vi "Z_ROI_compiler.vi"(7 "dISABLE":bool=TRUE, 8 "error in (no error)":errorcluster, 10 "Acquired z-plane index / volume index":i32, 11 "AOL_Globals":T2={"Imaging Protocol"=enum."AOL Z-Stack", "Number of POI"=0, "Number of Miniscans"=0, "Number of Trials"=0, "Number of Cycles "=0, "# Averaged Frames"=0, "Laser power (%)"=0, "Pockels"=0.0, "Acquisition Length (sec)"=0.0, "Fill time (us)"=0.0, "POI Dwell time (us)"=0.0, "Miniscan Dwell time per pixel (us)"=0.0, "PMT 1"=0.0, "PMT 2"=0.0, "Back Apperture"=200.0, "Frame Size"=0, "Center Frequency"=0.0, "Field of View"=0.0, "DwellTime (us)"=0.0, "Wavelength (nm)"=0.0, "Zoom"=0.0, "AOL Z"=0.0, "AOL Mode"=enum."Raster", "GridXY"=0.0, "GridZ"=0.0, "TriggerPeriod (sec)"=0.0, "Number of Pixels in Miniscan"=0, "Experiment folder path"=path "", "X centre"=0.0, "Y centre"=0.0, "Angle (degrees)"=0.0, "Plane Mode"=0, "Threshold"=[], "Regenerate Chirps"=FALSE, "Rectangle ROI length (pixels)"=0, "Rectangle ROI height (pixels)"=0, "AOD fill"=0, "Samples Wait after Trigger"=0, "StartUp Delay"=0, "Slip Cycle"=163840, "Add Cycle"=FALSE} {"Plane Mode" items=["XY Plane"]; "Frame Size" items=["100X100"=100, "128X128"=128, "200X200"=200, "256X256"=256, "512X512"=512, "1024x1024"=1024, "2048x2048"=2048]; "Back Apperture" format="%#.6g"; "Pockels" format="%#.6g"; "PMT 2" format="%#.6g"; "PMT 1" format="%#.6g"; "Angle (degrees)" format="%#.6g"; "POI Dwell time (us)" format="%#.6g"}) -> (0 "error out":errorcluster, 1 "AOL_Globals":T2={"Imaging Protocol"=enum."AOL Z-Stack", "Number of POI"=0, "Number of Miniscans"=0, "Number of Trials"=0, "Number of Cycles "=0, "# Averaged Frames"=0, "Laser power (%)"=0, "Pockels"=0.0, "Acquisition Length (sec)"=0.0, "Fill time (us)"=0.0, "POI Dwell time (us)"=0.0, "Miniscan Dwell time per pixel (us)"=0.0, "PMT 1"=0.0, "PMT 2"=0.0, "Back Apperture"=200.0, "Frame Size"=0, "Center Frequency"=0.0, "Field of View"=0.0, "DwellTime (us)"=0.0, "Wavelength (nm)"=0.0, "Zoom"=0.0, "AOL Z"=0.0, "AOL Mode"=enum."Raster", "GridXY"=0.0, "GridZ"=0.0, "TriggerPeriod (sec)"=0.0, "Number of Pixels in Miniscan"=0, "Experiment folder path"=path "", "X centre"=0.0, "Y centre"=0.0, "Angle (degrees)"=0.0, "Plane Mode"=0, "Threshold"=[], "Regenerate Chirps"=FALSE, "Rectangle ROI length (pixels)"=0, "Rectangle ROI height (pixels)"=0, "AOD fill"=0, "Samples Wait after Trigger"=0, "StartUp Delay"=0, "Slip Cycle"=163840, "Add Cycle"=FALSE} {"Plane Mode" items=["XY Plane"]; "Frame Size" items=["100X100"=100, "128X128"=128, "200X200"=200, "256X256"=256, "512X512"=512, "1024x1024"=1024, "2048x2048"=2048]; "Back Apperture" format="%#.6g"; "Pockels" format="%#.6g"; "PMT 2" format="%#.6g"; "PMT 1" format="%#.6g"; "Angle (degrees)" format="%#.6g"; "POI Dwell time (us)" format="%#.6g"}, 2 "ROI Coordinates (broken down to miniscans)":T7, 3 "Cycle time (us)":dbl, 4 "ROI Attributes (broken down to miniscans)":T1[](array[typedef]) {"ROI group ID" format="%#_6f"; "Laser Power (%)" format="%#_6f"; "Zoom" format="%#_6f"; "Frame Size" format="%#_6f"; "Number of lines" format="%#_6f"; "Composite ID" format="%#_6f"; "Angle (deg)" format="%#_6f"; "ROI Time (ns)" format="%#_6f"; "ROI ID" format="%#_6f"; "Pixels in ROI" format="%#_6f"; "ROI index" format="%#_6f"; "Z stop" format="%#_6f"; "Y stop" format="%#_6f"; "X stop" format="%#_6f"; "Z start" format="%#_6f"; "X start" format="%#_6f"; "Y start" format="%#_6f"}, 5 "Zoom":dbl[](array[numeric]), 6 "NO ROI AVAILABLE!!!":bool)   [LabVIEW 2013]
uses:
  Typedefs/ROI XY coordinates cluster.ctl
  Typedefs/Controls/AOL_Globals.ctl
  Typedefs/Imaging Protocols enum.ctl
  Typedefs/Frame Size.ctl
  Typedefs/AOL modes.ctl
  Typedefs/Plane Mode.ctl
  User Interface/Visualisation/Functional Imaging Viewer/Typedefs/ROI parameters data type.ctl
  User Interface/Visualisation/Functional Imaging Viewer/SubVIs/Experiment header interface/Typedefs/Save-Load-Save as-Load last enum.ctl
  User Interface/Visualisation/Functional Imaging Viewer/SubVIs/Experiment header interface/Typedefs/Header file type enum.ctl
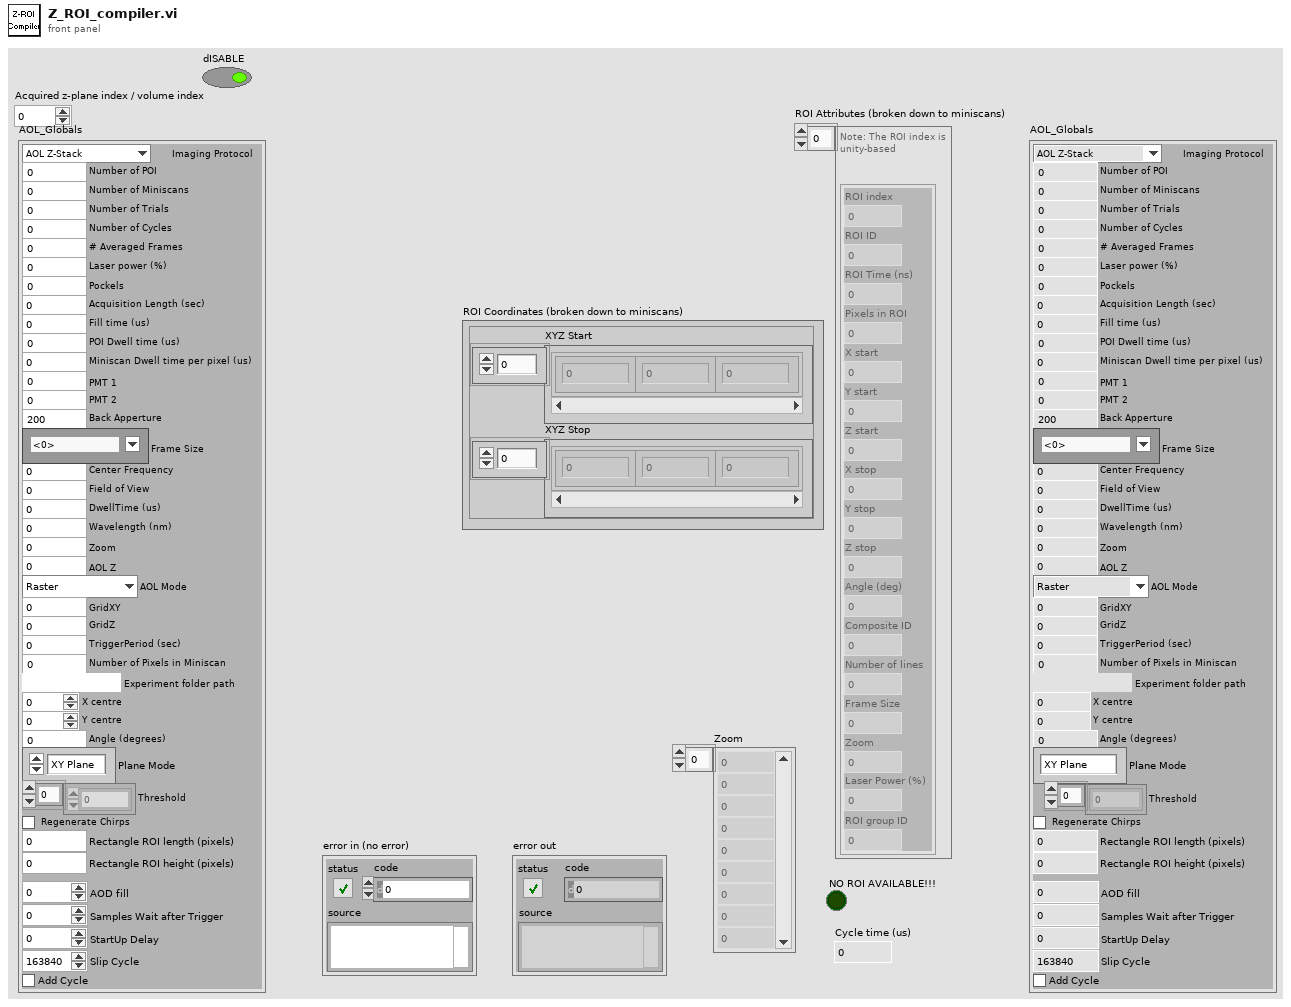
[diagram p1: front panel]
types:
  T1 = typedef "ROI parameters data type.ctl" = cluster{"ROI index":dbl, "ROI ID":dbl, "ROI Time (ns)":dbl, "Pixels in ROI":dbl, "X start":dbl, "Y start":dbl, "Z start":dbl, "X stop":dbl, "Y stop":dbl, "Z stop":dbl, "Angle (deg)":dbl, "Composite ID":dbl, "Number of lines":dbl, "Frame Size":dbl, "Zoom":dbl, "Laser Power (%)":dbl, "ROI group ID":dbl}
  T2 = typedef "AOL_Globals.ctl" = cluster{"Imaging Protocol":T3, "Number of POI":u16, "Number of Miniscans":u16, "Number of Trials":u16, "Number of Cycles ":u64, "# Averaged Frames":u16, "Laser power (%)":u8, "Pockels":dbl, "Acquisition Length (sec)":dbl, "Fill time (us)":dbl, "POI Dwell time (us)":dbl, "Miniscan Dwell time per pixel (us)":dbl, "PMT 1":dbl, "PMT 2":dbl, "Back Apperture":dbl, "Frame Size":T4, "Center Frequency":dbl, "Field of View":dbl, "DwellTime (us)":dbl, "Wavelength (nm)":dbl, "Zoom":dbl, "AOL Z":dbl, "AOL Mode":T5, "GridXY":dbl, "GridZ":dbl, "TriggerPeriod (sec)":dbl, "Number of Pixels in Miniscan":u16, "Experiment folder path":path, "X centre":dbl, "Y centre":dbl, "Angle (degrees)":dbl, "Plane Mode":T6, "Threshold":u16[], "Regenerate Chirps":bool, "Rectangle ROI length (pixels)":u16, "Rectangle ROI height (pixels)":u16, "AOD fill":u16, "Samples Wait after Trigger":u16, "StartUp Delay":i32, "Slip Cycle":u32, "Add Cycle":bool}
  T3 = typedef "Imaging Protocols enum.ctl" = enum16{"AOL Z-Stack", "Motor Z Stack", "Functional Acquisition", "Single Plane Acquisition", "Volume Acquisition", "Live Imaging", "Live Plane Imaging", "Live Volume Imaging"}
  T4 = typedef "Frame Size.ctl" = u16
  T5 = typedef "AOL modes.ctl" = enum16{"Raster", "Structural", "Pointing", "Mini Scan", "Alignment"}
  T6 = typedef "Plane Mode.ctl" = u16
  T7 = typedef "ROI XY coordinates cluster.ctl" = cluster{"XYZ Start":cluster{"X":sgl, "Y":sgl, "Z":sgl}[], "XYZ Stop":cluster{"X":sgl, "Y":sgl, "Z":sgl}[]}
  T8 = typedef "Header file type enum.ctl" = enum16{"All parameters", "Params for funct acq w ROI or mscn", "Params for funct acq w rectangles", "Live imaging header parameters", "AOL Parameters"}
  T9 = typedef "Save-Load-Save as-Load last enum.ctl" = enum16{"Save file", "Save file as", "Load file", "Load last file"}
  T10 = typedef "Header parameters cluster-ALL.ctl" = cluster{"Imaging Protocol":T3, "Number of POI":u16, "Number of Miniscans":u16, "Number of Trials":u16, "Number of Cycles ":u64, "# Averaged Frames":u16, "Laser power (%)":u8, "Pockels":dbl, "Acquisition Length (sec)":dbl, "Fill time (us)":dbl, "POI Dwell time (us)":dbl, "Miniscan Dwell time per pixel (us)":dbl, "PMT 1":dbl, "PMT 2":dbl, "Back Apperture":dbl, "Zoom":dbl, "Frame Size":T4, "Center Frequency":dbl, "Field of View":dbl, "DwellTime (us)":dbl, "Wavelength (nm)":dbl, "AOL Z":dbl, "AOL Mode":T5, "GridXY":dbl, "GridZ":dbl, "TriggerDelay (sec)":dbl, "Number of Pixels in Miniscan":u16, "Experiment folder path":path, "X centre":dbl, "Y centre":dbl, "Angle (degrees)":dbl, "Plane Mode":T6, "Software version":dbl, "Objective":T11, "MotorZ Calibration":u32, "Pockels Calibration":u32, "Threshold":u16[], "Video length (sec)":dbl, "Frame rate (fps)":u8, "Rectangle ROI length (pixels)":u16, "Rectangle ROI height (pixels)":u16}
  T11 = typedef "Objective selector control enum.ctl" = string
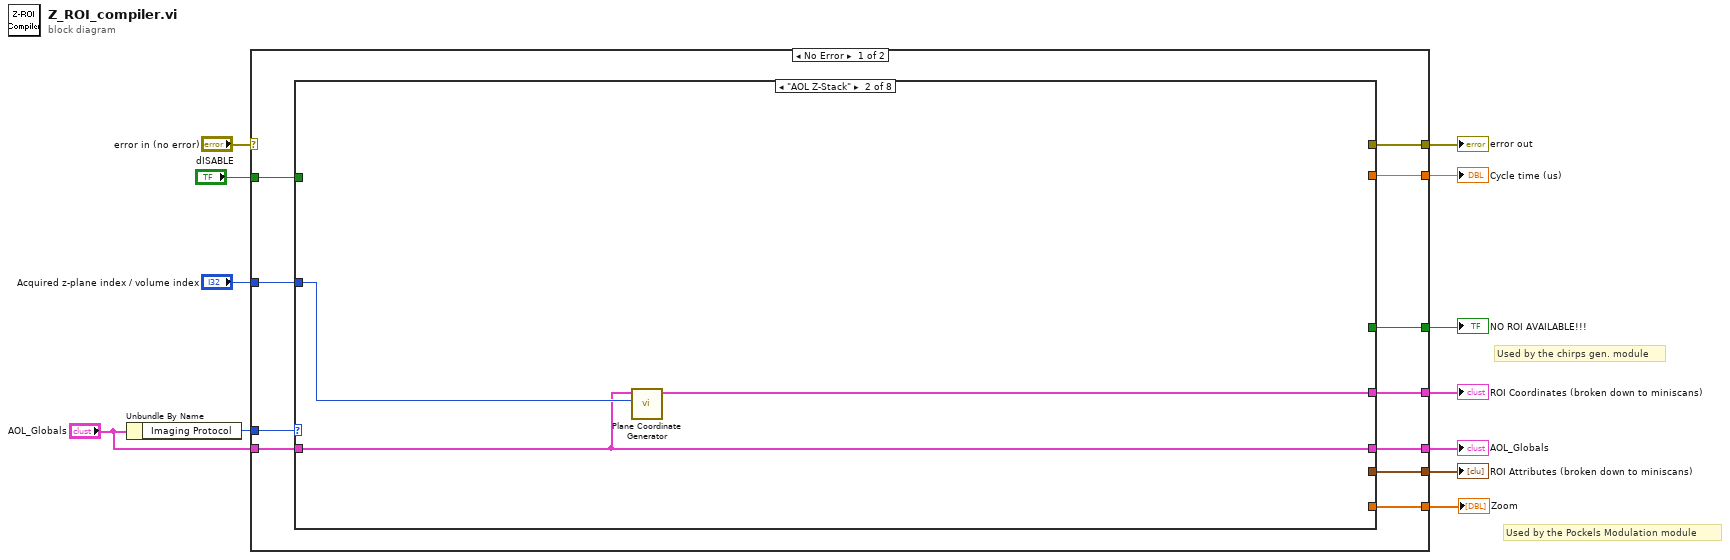
[diagram p0: block diagram]
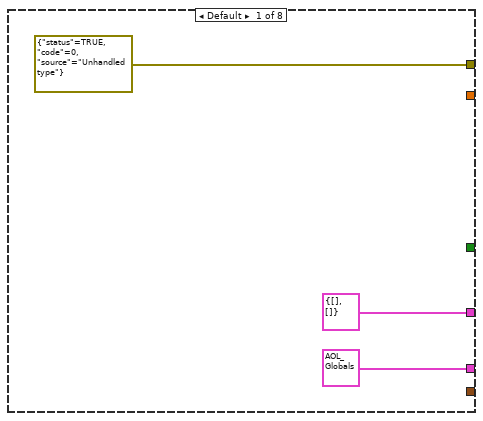
[diagram p2: hidden frame]
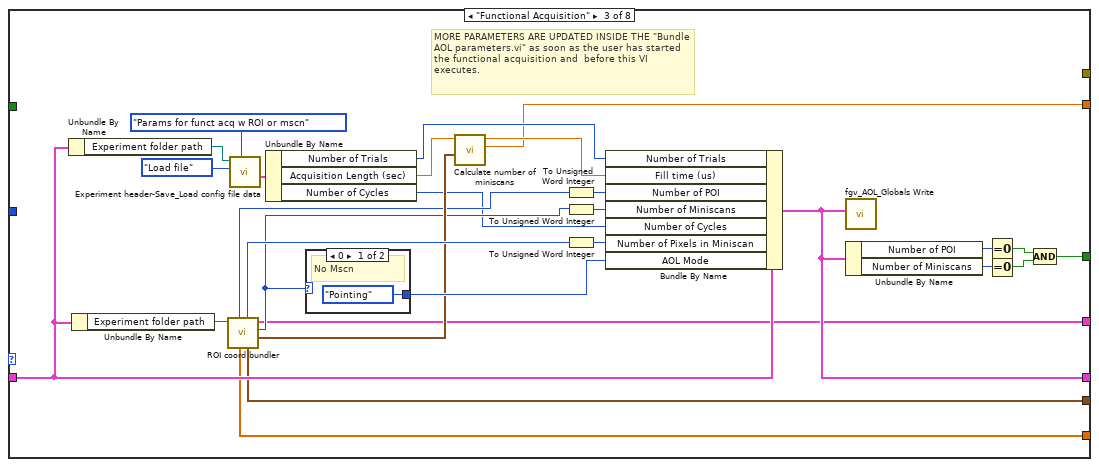
[diagram p3: hidden frame]
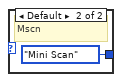
[diagram p4: hidden frame]
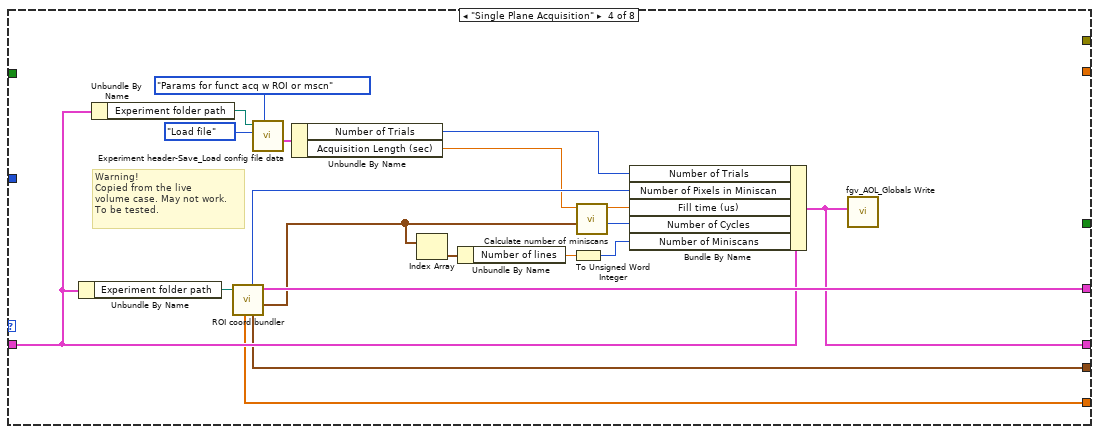
[diagram p5: hidden frame]
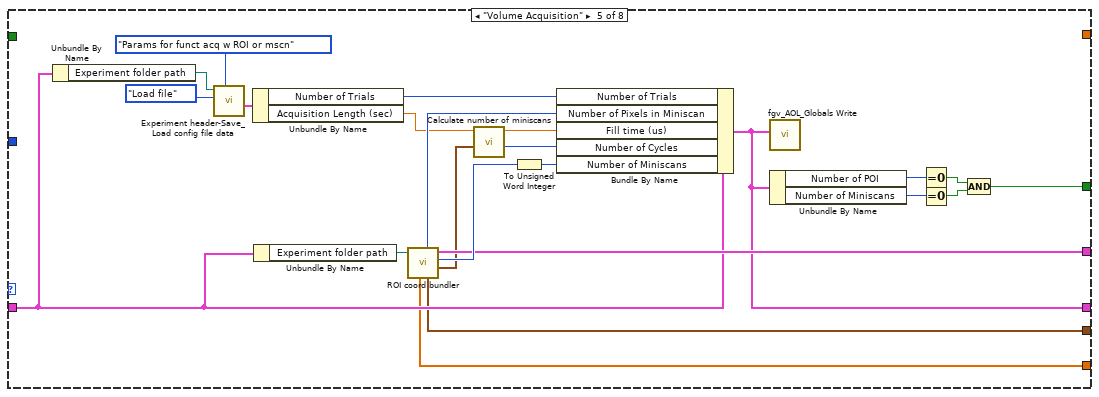
[diagram p6: hidden frame]
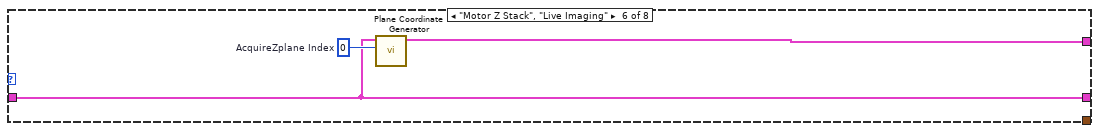
[diagram p7: hidden frame]
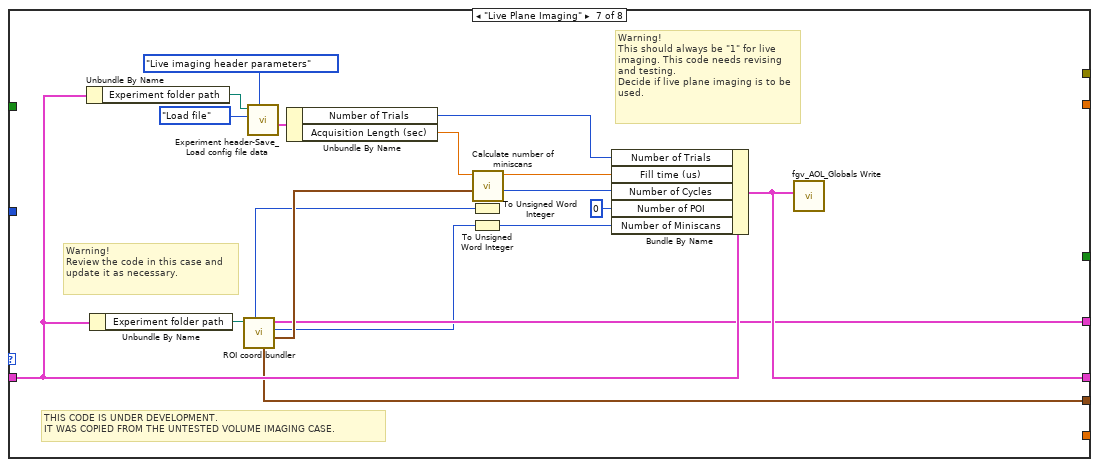
[diagram p8: hidden frame]
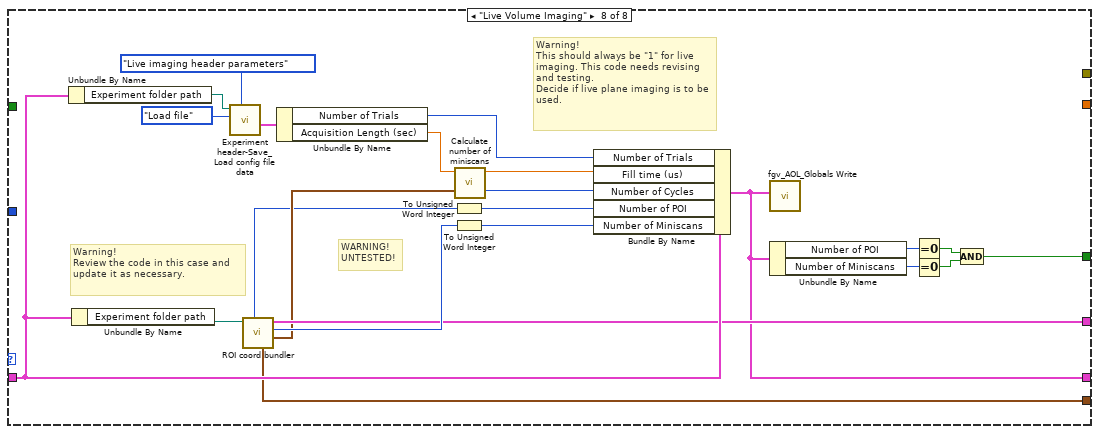
[diagram p9: hidden frame]
diagram:
  # "Used by the Pockels Modulation module"
  # "Used by the chirps gen. module"
  n1 = Unbundle By Name("AOL_Globals") -> ("Imaging Protocol"=w10:T3)
  n2 = case shown="No Error" "error in (no error)" {
    selector: "error in (no error)" -> [_ w146]
    tunnel: "Acquired z-plane index / volume index" -> [w23 _]
    tunnel: [w22 _] -> w11
    tunnel: w10 -> [w21 _]
    tunnel: [w20 w146] -> w9
    tunnel: "AOL_Globals" -> [w19 _]
    tunnel: [w18 _] -> w3
    tunnel: [w17 _] -> w6
    tunnel: [w16 _] -> w5
    tunnel: [w15 _] -> w4
    tunnel: [w14 _] -> w2
    tunnel: "dISABLE" -> [w13 _]
    frame No Error {
      n3 = case shown="\"AOL Z-Stack\"" w21 {
        tunnel: [T7 {"XYZ Start"=[], "XYZ Stop"=[]} ("miniScan_Coordinates") w28 w31 w74 w96 w103 w110 w133] -> w22
        tunnel: w23 -> [_ w29 _ _ _ _ _ _]
        tunnel: w19 -> [_ w27 w51 w63 w81 w102 w115 w137]
        tunnel: [errorcluster {"status"=TRUE, "code"=0, "source"="Unhandled type"} ("error out") _ _ _ _ _ _ _] -> w20
        tunnel: [T2 {"Imaging Protocol"=enum."AOL Z-Stack", "Number of POI"=0, "Number of Miniscans"=0, "Number of Trials"=0, "Number of Cycles "=0, "# Averaged Frames"=0, "Laser power (%)"=0, "Pockels"=0.0, "Acquisition Length (sec)"=0.0, "Fill time (us)"=0.0, "POI Dwell time (us)"=0.0, "Miniscan Dwell time per pixel (us)"=0.0, "PMT 1"=0.0, "PMT 2"=0.0, "Back Apperture"=200.0, "Frame Size"=0, "Center Frequency"=0.0, "Field of View"=0.0, "DwellTime (us)"=0.0, "Wavelength (nm)"=0.0, "Zoom"=0.0, "AOL Z"=0.0, "AOL Mode"=enum."Raster", "GridXY"=0.0, "GridZ"=0.0, "TriggerPeriod (sec)"=0.0, "Number of Pixels in Miniscan"=0, "Experiment folder path"=path "", "X centre"=0.0, "Y centre"=0.0, "Angle (degrees)"=0.0, "Plane Mode"=0, "Threshold"=[], "Regenerate Chirps"=FALSE, "Rectangle ROI length (pixels)"=0, "Rectangle ROI height (pixels)"=0, "AOD fill"=0, "Samples Wait after Trigger"=0, "StartUp Delay"=0, "Slip Cycle"=0, "Add Cycle"=FALSE} ("AOL_Globals") w27 w41 w65 w83 w102 w113 w126] -> w18
        tunnel: [_ _ w36 _ _ _ _ _] -> w17
        tunnel: [_ _ w32 w60 w80 _ w106 w123] -> w16
        tunnel: [_ _ w30 w61 w79 _ _ _] -> w15
        tunnel: [_ _ w40 _ w82 _ _ w125] -> w14
        tunnel: w13 -> [_ _ _ _ _ _ _ _]
        frame Default {
        }
        frame "AOL Z-Stack" {
          n4 = call "Plane Coordinate Generator.vi"("AcquireZplane Index"=w29, "AOL_Globals"=w27) -> ("ROI Attributes (broken down to miniscans)"=w28:T7)  [unwired: 8 in, 1 out]
        }
        frame "Functional Acquisition" {
          # "MORE PARAMETERS ARE UPDATED INSIDE THE \"Bundle AOL parameters.vi\" as soon as the user has started the functional acquisition and  before this VI executes."
          n5 = Unbundle By Name(w51) -> ("Experiment folder path"=w55:path)
          n6 = Unbundle By Name(w51) -> ("Experiment folder path"=w49:path)
          n7 = call "ROI coord bundler.vi"("Experiment folder path"=w49) -> ("ROI Attributes"=w38:T1[], "Total number of miniscans"=w34:i32, "ROI Coordinates (broken down to miniscans)"=w31:T7, "ROI Attributes (broken down to miniscans)"=w32:T1[], "Number of pixels in single miniscan"=w48:i32, "Zoom"=w30:dbl[], "Number of POIs"=w35:i32)  [unwired: 3 in, 1 out]
          n8 = call "Experiment header-Save_Load config file data.vi"("Header file type"=Header_file_type_enum."Params for funct acq w ROI or mscn", "Function"=Save-Load-Save_as-Load_last_enum."Load file", "Experiment data folder path"=w55) -> ("All header parameters out"=w53:T10)  [unwired: 7 in, 1 out]
          n9 = Unbundle By Name(w53) -> ("Number of Trials"=w37:u16, "Acquisition Length (sec)"=w52:dbl, "Number of Cycles"=w33:u64)
          n10 = case shown="0" w34 {
            tunnel: [AOL_modes."Pointing" ("AOL Mode") AOL_modes."Mini Scan" ("AOL Mode")] -> w46
            frame 0 {
              # "No Mscn"
            }
            frame Default {
              # "Mscn"
            }
          }
          n11 = call "Calculate number of miniscans.vi"("XYZ Coordinates"=w38, "Acquisition length (sec)"=w52) -> ("Cycle time (us)"=w36:dbl, "AOD fill time (us)"=w57:dbl)  [unwired: 7 in, 1 out]
          n12 = To Unsigned Word Integer(number=w35) -> (unsigned 16bit integer=w56:u16)
          n13 = To Unsigned Word Integer(number=w34) -> (unsigned 16bit integer=w47:u16)
          n14 = To Unsigned Word Integer(number=w48) -> (unsigned 16bit integer=w39:u16)
          n15 = Bundle By Name(cluster=w51, "Number of Trials"=w37, "Fill time (us)"=w57, "Number of POI"=w56, "Number of Miniscans"=w47, "Number of Cycles"=w33, "Number of Pixels in Miniscan"=w39, "AOL Mode"=w46) -> (w41:T2)
          n16 = call "fgv_AOL_Globals Write.vi"("AOL_Globals"=w41) -> ()  [unwired: 10 in, 1 out]
          n17 = Unbundle By Name(w41) -> ("Number of POI"=w44:u16, "Number of Miniscans"=w45:u16)
          n18 = Equal To 0?(x=w44) -> (x = 0?=w43:bool)
          n19 = Equal To 0?(x=w45) -> (x = 0?=w42:bool)
          n20 = Compound Arithmetic op=AND(w43, w42) -> (w40:bool)
        }
        frame "Single Plane Acquisition" {
          # "Warning!\nCopied from the live\nvolume case. May not work.\nTo be tested."
          n21 = Unbundle By Name(w63) -> ("Experiment folder path"=w75:path)
          n22 = Unbundle By Name(w63) -> ("Experiment folder path"=w72:path)
          n23 = call "ROI coord bundler.vi"("Experiment folder path"=w75) -> ("ROI Attributes"=w62:T1[], "ROI Coordinates (broken down to miniscans)"=w74:T7, "ROI Attributes (broken down to miniscans)"=w60:T1[], "Number of pixels in single miniscan"=w73:i32, "Zoom"=w61:dbl[])  [unwired: 3 in, 3 out]
          n24 = call "Experiment header-Save_Load config file data.vi"("Header file type"=Header_file_type_enum."Params for funct acq w ROI or mscn", "Function"=Save-Load-Save_as-Load_last_enum."Load file", "Experiment data folder path"=w72) -> ("All header parameters out"=w70:T10)  [unwired: 7 in, 1 out]
          n25 = Unbundle By Name(w70) -> ("Number of Trials"=w68:u16, "Acquisition Length (sec)"=w69:dbl)
          n26 = Index Array(array=w62) -> (element=w67:T1)  [unwired: 1 in]
          n27 = Unbundle By Name(w67) -> ("Number of lines"=w66:dbl)
          n28 = To Unsigned Word Integer(number=w66) -> (unsigned 16bit integer=w77:u16)
          n29 = call "Calculate number of miniscans.vi"("XYZ Coordinates"=w62, "Acquisition length (sec)"=w69) -> ("Number of cycles"=w76:u64, "AOD fill time (us)"=w78:dbl)  [unwired: 7 in, 1 out]
          n30 = Bundle By Name(cluster=w63, "Number of Trials"=w68, "Number of Pixels in Miniscan"=w73, "Fill time (us)"=w78, "Number of Cycles"=w76, "Number of Miniscans"=w77) -> (w65:T2)
          n31 = call "fgv_AOL_Globals Write.vi"("AOL_Globals"=w65) -> ()  [unwired: 10 in, 1 out]
        }
        frame "Volume Acquisition" {
          n32 = Unbundle By Name(w81) -> ("Experiment folder path"=w94:path)
          n33 = call "Experiment header-Save_Load config file data.vi"("Header file type"=Header_file_type_enum."Params for funct acq w ROI or mscn", "Function"=Save-Load-Save_as-Load_last_enum."Load file", "Experiment data folder path"=w94) -> ("All header parameters out"=w92:T10)  [unwired: 7 in, 1 out]
          n34 = Unbundle By Name(w92) -> ("Number of Trials"=w90:u16, "Acquisition Length (sec)"=w91:dbl)
          n35 = Unbundle By Name(w81) -> ("Experiment folder path"=w98:path)
          n36 = call "ROI coord bundler.vi"("Experiment folder path"=w98) -> ("ROI Attributes"=w88:T1[], "Total number of miniscans"=w97:i32, "ROI Coordinates (broken down to miniscans)"=w96:T7, "ROI Attributes (broken down to miniscans)"=w80:T1[], "Number of pixels in single miniscan"=w95:i32, "Zoom"=w79:dbl[])  [unwired: 3 in, 2 out]
          n37 = call "Calculate number of miniscans.vi"("XYZ Coordinates"=w88, "Acquisition length (sec)"=w91) -> ("Number of cycles"=w99:u64, "AOD fill time (us)"=w101:dbl)  [unwired: 7 in, 1 out]
          n38 = To Unsigned Word Integer(number=w97) -> (unsigned 16bit integer=w100:u16)
          n39 = Bundle By Name(cluster=w81, "Number of Trials"=w90, "Number of Pixels in Miniscan"=w95, "Fill time (us)"=w101, "Number of Cycles"=w99, "Number of Miniscans"=w100) -> (w83:T2)
          n40 = call "fgv_AOL_Globals Write.vi"("AOL_Globals"=w83) -> ()  [unwired: 10 in, 1 out]
          n41 = Unbundle By Name(w83) -> ("Number of POI"=w86:u16, "Number of Miniscans"=w87:u16)
          n42 = Equal To 0?(x=w86) -> (x = 0?=w85:bool)
          n43 = Equal To 0?(x=w87) -> (x = 0?=w84:bool)
          n44 = Compound Arithmetic op=AND(w85, w84) -> (w82:bool)
        }
        frame "Motor Z Stack", "Live Imaging" {
          w104 = 0  # AcquireZplane Index
          n45 = call "Plane Coordinate Generator.vi"("AcquireZplane Index"=w104, "AOL_Globals"=w102) -> ("ROI Attributes (broken down to miniscans)"=w103:T7)  [unwired: 8 in, 1 out]
        }
        frame "Live Plane Imaging" {
          # "Warning!\nThis should always be \"1\" for live imaging. This code needs revising and testing.\nDecide if live plane imaging is to be used."
          # "THIS CODE IS UNDER DEVELOPMENT.\nIT WAS COPIED FROM THE UNTESTED VOLUME IMAGING CASE."
          # "Warning!\nReview the code in this case and update it as necessary."
          n46 = Unbundle By Name(w115) -> ("Experiment folder path"=w119:path)
          n47 = Unbundle By Name(w115) -> ("Experiment folder path"=w109:path)
          n48 = call "ROI coord bundler.vi"("Experiment folder path"=w109) -> ("ROI Attributes"=w111:T1[], "Total number of miniscans"=w108:i32, "ROI Coordinates (broken down to miniscans)"=w110:T7, "ROI Attributes (broken down to miniscans)"=w106:T1[], "Number of POIs"=w107:i32)  [unwired: 3 in, 3 out]
          n49 = call "Experiment header-Save_Load config file data.vi"("Header file type"=Header_file_type_enum."Live imaging header parameters", "Function"=Save-Load-Save_as-Load_last_enum."Load file", "Experiment data folder path"=w119) -> ("All header parameters out"=w117:T10)  [unwired: 7 in, 1 out]
          n50 = Unbundle By Name(w117) -> ("Number of Trials"=w114:u16, "Acquisition Length (sec)"=w116:dbl)
          n51 = To Unsigned Word Integer(number=w107) -> ()  [unwired: 1 out]
          n52 = To Unsigned Word Integer(number=w108) -> (unsigned 16bit integer=w121:u16)
          n53 = call "Calculate number of miniscans.vi"("XYZ Coordinates"=w111, "Acquisition length (sec)"=w116) -> ("Number of cycles"=w120:u64, "AOD fill time (us)"=w122:dbl)  [unwired: 7 in, 1 out]
          n54 = Bundle By Name(cluster=w115, "Number of Trials"=w114, "Fill time (us)"=w122, "Number of Cycles"=w120, "Number of POI"=u16 0, "Number of Miniscans"=w121) -> (w113:T2)
          n55 = call "fgv_AOL_Globals Write.vi"("AOL_Globals"=w113) -> ()  [unwired: 10 in, 1 out]
        }
        frame "Live Volume Imaging" {
          # "Warning!\nThis should always be \"1\" for live imaging. This code needs revising and testing.\nDecide if live plane imaging is to be used."
          # "WARNING!\nUNTESTED!"
          # "Warning!\nReview the code in this case and update it as necessary."
          n56 = Unbundle By Name(w137) -> ("Experiment folder path"=w141:path)
          n57 = Unbundle By Name(w137) -> ("Experiment folder path"=w132:path)
          n58 = call "Experiment header-Save_Load config file data.vi"("Header file type"=Header_file_type_enum."Live imaging header parameters", "Function"=Save-Load-Save_as-Load_last_enum."Load file", "Experiment data folder path"=w141) -> ("All header parameters out"=w139:T10)  [unwired: 7 in, 1 out]
          n59 = call "ROI coord bundler.vi"("Experiment folder path"=w132) -> ("ROI Attributes"=w131:T1[], "Total number of miniscans"=w134:i32, "ROI Coordinates (broken down to miniscans)"=w133:T7, "ROI Attributes (broken down to miniscans)"=w123:T1[], "Number of POIs"=w124:i32)  [unwired: 3 in, 3 out]
          n60 = Unbundle By Name(w139) -> ("Number of Trials"=w136:u16, "Acquisition Length (sec)"=w138:dbl)
          n61 = To Unsigned Word Integer(number=w124) -> (unsigned 16bit integer=w144:u16)
          n62 = To Unsigned Word Integer(number=w134) -> (unsigned 16bit integer=w143:u16)
          n63 = call "Calculate number of miniscans.vi"("XYZ Coordinates"=w131, "Acquisition length (sec)"=w138) -> ("Number of cycles"=w142:u64, "AOD fill time (us)"=w145:dbl)  [unwired: 7 in, 1 out]
          n64 = Bundle By Name(cluster=w137, "Number of Trials"=w136, "Fill time (us)"=w145, "Number of Cycles"=w142, "Number of POI"=w144, "Number of Miniscans"=w143) -> (w126:T2)
          n65 = call "fgv_AOL_Globals Write.vi"("AOL_Globals"=w126) -> ()  [unwired: 10 in, 1 out]
          n66 = Unbundle By Name(w126) -> ("Number of POI"=w129:u16, "Number of Miniscans"=w130:u16)
          n67 = Equal To 0?(x=w129) -> (x = 0?=w128:bool)
          n68 = Equal To 0?(x=w130) -> (x = 0?=w127:bool)
          n69 = Compound Arithmetic op=AND(w128, w127) -> (w125:bool)
        }
      }
    }
    frame Error {
    }
  }
  "ROI Coordinates (broken down to miniscans)" <- w11
  "error out" <- w9
  "AOL_Globals" <- w3
  "Cycle time (us)" <- w6
  "ROI Attributes (broken down to miniscans)" <- w5
  "Zoom" <- w4
  "NO ROI AVAILABLE!!!" <- w2
